vi "tastierino.vi"() -> ()   [LabVIEW 2017]
panel:
  in  "OK Button 2":bool
  out "OUTPUT":string
  in  ",":bool
  out "Numeric":dbl format="%#.10f"
  in  "Cancel Button":bool
  in  "Boolean 4":bool
  in  "Boolean 3":bool
  in  "Boolean 2":bool
  in  "Boolean":bool
  out "TEMP":string
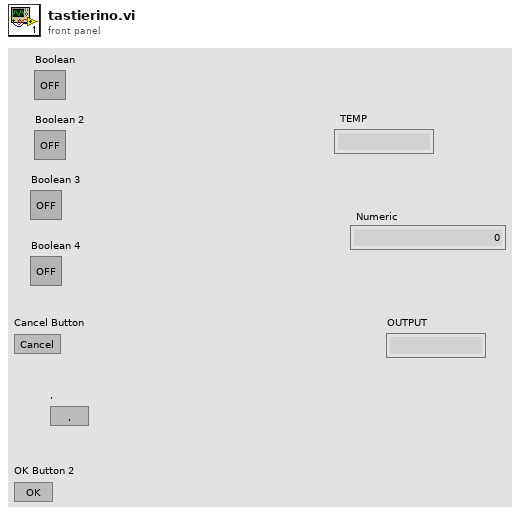
[diagram p1: front panel]
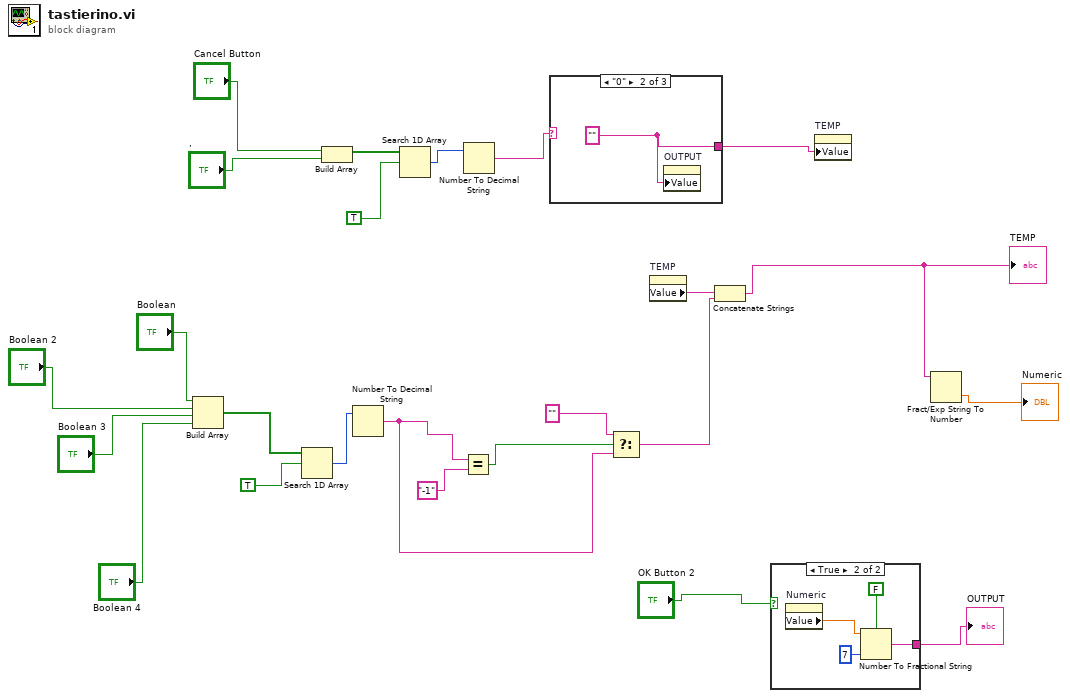
[diagram p0: block diagram]
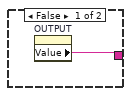
[diagram p2: hidden frame]
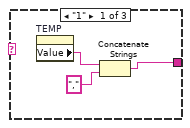
[diagram p3: hidden frame]
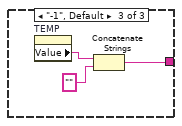
[diagram p4: hidden frame]
diagram:
  n1 = Build Array("Boolean", "Boolean 2", "Boolean 3", "Boolean 4") -> (w24:bool[])
  n2 = Search 1D Array(1D array=w24, element=TRUE) -> (index of element=w17:i32)  [unwired: 1 in]
  n3 = Build Array("Cancel Button", ",") -> (w4:bool[])
  n4 = Number To Decimal String(number=w17) -> (decimal integer string=w19:string)  [unwired: 1 in]
  n5 = Search 1D Array(1D array=w4, element=TRUE) -> (index of element=w5:i32)  [unwired: 1 in]
  n6 = Equal?(x=w19, y="-1") -> (x = y?=w18:bool)
  n7 = Number To Decimal String(number=w5) -> (decimal integer string=w6:string)  [unwired: 1 in]
  n8 = case shown="\"0\"" w6 {
    tunnel: [w26 w28 w30] -> w9
    frame "1" {
      n9 = property on="TEMP" class="Str"() -> ("Value"=w27:string)  [unwired: 2 in, 2 out]
      n10 = Concatenate Strings(w27, "," ("string")) -> (w26:string)
    }
    frame "0" {
      w28 = ""
      n11 = property on="OUTPUT" class="Str"("Value"=w28) -> ()  [unwired: 2 in, 2 out]
    }
    frame "-1", Default {
      n12 = property on="TEMP" class="Str"() -> ("Value"=w31:string)  [unwired: 2 in, 2 out]
      n13 = Concatenate Strings(w31, "" ("string")) -> (w30:string)
    }
  }
  n14 = Select(t="" ("f"), s=w18, f=w19) -> (s? t:f=w13:string)
  n15 = property on="TEMP" class="Str"() -> ("Value"=w10:string)  [unwired: 2 in, 2 out]
  n16 = Concatenate Strings(w10, w13) -> (w11:string)
  "TEMP" <- w11
  n17 = case shown="True" "OK Button 2" {
    tunnel: [w32 w33] -> w1
    frame False {
      n18 = property on="OUTPUT" class="Str"() -> ("Value"=w32:string)  [unwired: 2 in, 2 out]
    }
    frame True {
      n19 = property on="Numeric" class="DigNum (strict)"() -> ("Value"=w36:dbl)  [unwired: 2 in, 2 out]
      n20 = Number To Fractional String(use system decimal point (T)=FALSE, number=w36, precision (6)=i16 7) -> (F-format string=w33:string)  [unwired: 1 in]
    }
  }
  "OUTPUT" <- w1
  n21 = property on="TEMP" class="Str"("Value"=w9) -> ()  [unwired: 2 in, 2 out]
  n22 = Fract/Exp String To Number(string=w11) -> (number=→"Numeric":dbl)  [unwired: 3 in, 1 out]
